vi "gimbale.vi"(11 "GIMBAL":refnum<visa-resource-name>) -> ()   [LabVIEW 2014]
uses:
  <vilib>/Instr/_visa.llb/VISA Configure Serial Port (Instr).vi
panel:
  in  "GÓRA 3":bool caption="GÓRA"
  in  "Dӣ 3":bool caption="Dӣ"
  in  "PRAWO 3":bool caption="PRAWO"
  in  "LEWO 3":bool caption="LEWO"
  in  "LEWO 2":bool caption="LEWO"
  in  "PRAWO 2":bool caption="PRAWO"
  in  "stop":bool
  in  "Dӣ":bool
  in  "PRAWO":bool
  in  "LEWO":bool
  in  "GÓRA":bool
  # "sterowanie drugim dużym gimbalem\n(skonfigurowany na trzecim adresie*)\n\n*gimbal do skonfigurowania wg polecenia\nna diagramie"
  # "sterowanie gimbalem dużym\n(skonfigurowany na pierwszym adresie)"
  # "sterowanie gimbalem małym\n(skonfigurowany na drugim adresie)"
  # "UWAGA!\nZatrzymywać program STOPem"
  # "Oba gimbale działają na jednym porcie\nUstawić port, na którym widziany jest RS485"
  # "W zależności jak długo jest wciśnięty przycisk, tak długo wykonywany jest ruch gimbalal; \npuszczając przycisk, gimbal przestaje wykonywać ruch; \nnie można wykonywać dwóch ruchów równocześnie na jednym gimbalu;"
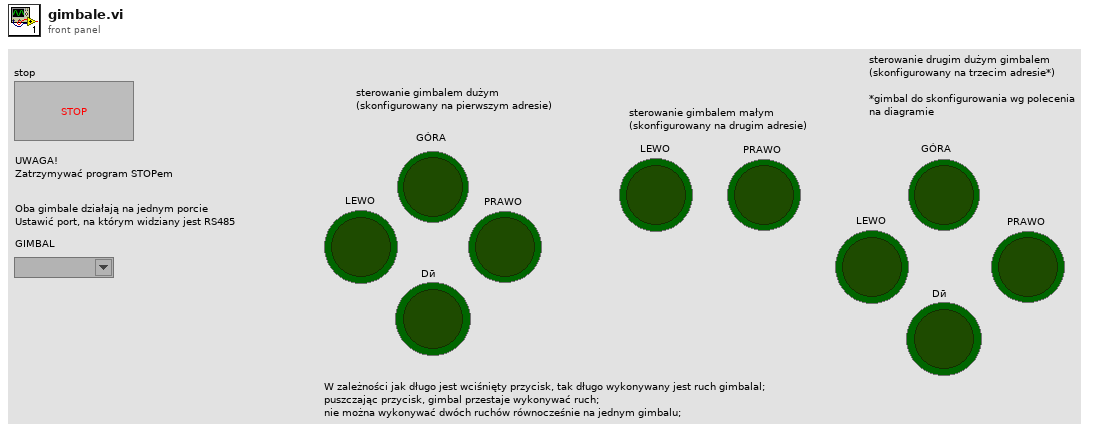
[diagram p1: front panel]
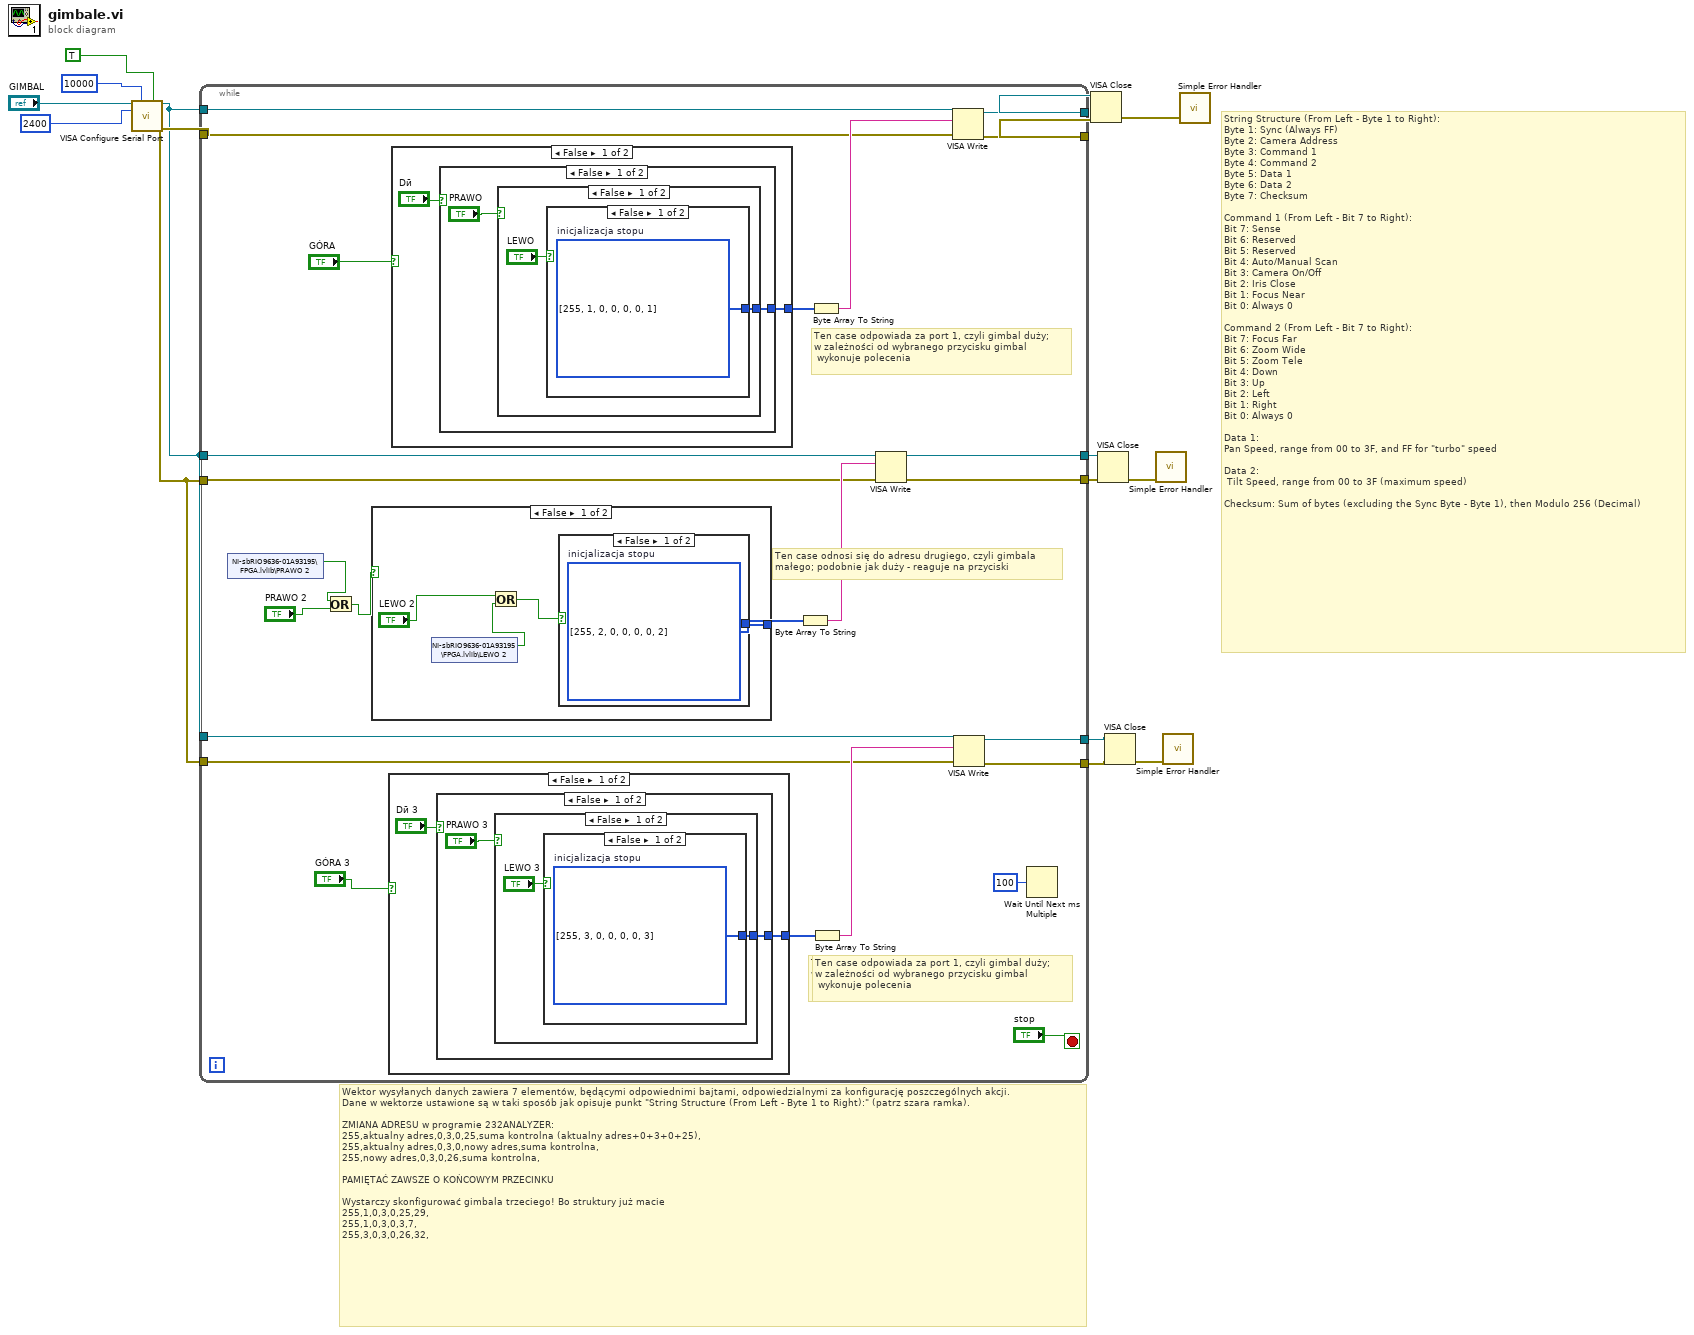
[diagram p0: block diagram]
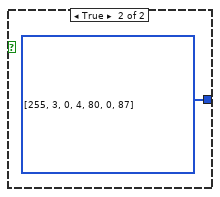
[diagram p2: hidden frame]
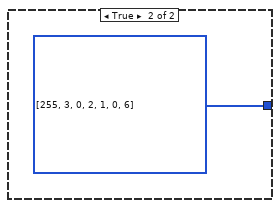
[diagram p3: hidden frame]
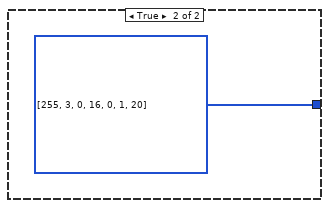
[diagram p4: hidden frame]
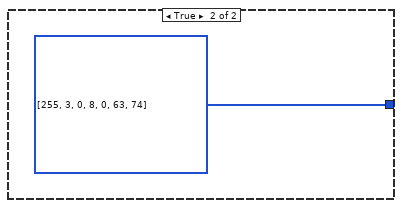
[diagram p5: hidden frame]
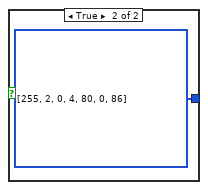
[diagram p6: hidden frame]
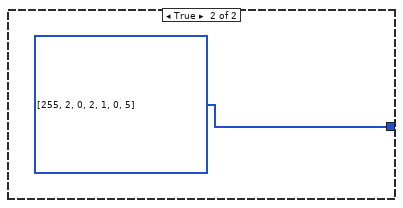
[diagram p7: hidden frame]
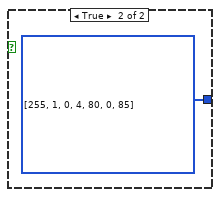
[diagram p8: hidden frame]
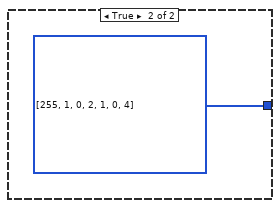
[diagram p9: hidden frame]
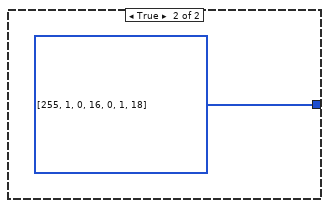
[diagram p10: hidden frame]
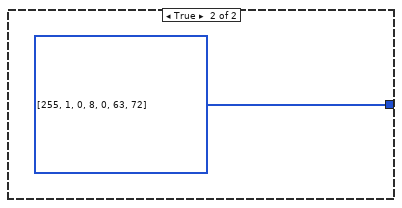
[diagram p11: hidden frame]
diagram:
  # "Wektor wysyłanych danych zawiera 7 elementów, będącymi odpowiednimi bajtami, odpowiedzialnymi za konfigurację poszczególnych akcji.\nDane w wektorze ustawione są w taki sposób jak opisuje punkt \"String Structure (From Left - Byte 1 to Right):\" (patrz szara ramka).\n\nZMIANA ADRESU w programie 232ANALYZER:\n255,aktualny adres,0,3,0,25,suma kontrolna (aktualny adres+0+3+0+25),\n255,aktualny adres,0,3,0,nowy adres,suma kontrolna,\n255,nowy adres,0,3,0,26,suma kontrolna,\n\nPAMIĘTAĆ ZAWSZE O KOŃCOWYM PRZECINKU\n\nWystarczy skonfigurować gimbala trzeciego! Bo struktury już macie\n255,1,0,3,0,25,29,\n255,1,0,3,0,3,7,\n255,3,0,3,0,26,32,"
  # "String Structure (From Left - Byte 1 to Right):\nByte 1: Sync (Always FF)\nByte 2: Camera Address\nByte 3: Command 1\nByte 4: Command 2\nByte 5: Data 1\nByte 6: Data 2\nByte 7: Checksum\n\nCommand 1 (From Left - Bit 7 to Right):\nBit 7: Sense\nBit 6: Reserved\nBit 5: Reserved\nBit 4: Auto/Manual Scan\nBit 3: Camera On/Off\nBit 2: Iris Close\nBit 1: Focus Near\nBit 0: Always 0\n\nCommand 2 (From Left - Bit 7 to Right):\nBit 7: Focus Far\nBit 6: Zoom Wide\nBit 5: Zoom Tele\nBit 4: Down\nBit 3: Up\nBit 2: Left\nBit 1: Right\nBit 0: Always 0\n\nData 1:\nPan Speed, range from 00 to 3F, and FF for \"turbo\" speed\n\nData 2:\n Tilt Speed, range from 00 to 3F (maximum speed)\n\nChecksum: Sum of bytes (excluding the Sync Byte - Byte 1), then Modulo 256 (Decimal)"
  n1 = call-poly "VISA Configure Serial Port"("VISA resource name"="GIMBAL", "timeout (10sec)"=u32 10000, "Enable Termination\nChar (T)"=TRUE ("Enable Termination\nChar (T)"), "baud rate (9600)"=u32 2400) -> ("VISA resource name out"=w1:refnum<visa-resource-name>, "error out"=w2:errorcluster)  [unwired: 10 in]
  n2 = while {
    tunnel: w2 -> [w37]
    tunnel: [w36] -> w10
    tunnel: w1 -> [w35]
    tunnel: [w34] -> w9
    tunnel: [w30] -> w7
    tunnel: [w29] -> w6
    tunnel: w1 -> [w28]
    tunnel: w2 -> [w27]
    tunnel: [w25] -> w4
    tunnel: [w24] -> w3
    tunnel: w2 -> [w23]
    tunnel: w1 -> [w22]
    stop <- "stop" stop-if-true
    # "Ten case odpowiada za port 3, czyli gimbal duży;\nw zależności od wybranego przycisku gimbal\n wykonuje polecenia"
    # "Ten case odpowiada za port 1, czyli gimbal duży;\nw zależności od wybranego przycisku gimbal\n wykonuje polecenia"
    # "Ten case odnosi się do adresu drugiego, czyli gimbala \nmałego; podobnie jak duży - reaguje na przyciski"
    # "Ten case odpowiada za port 1, czyli gimbal duży;\nw zależności od wybranego przycisku gimbal\n wykonuje polecenia"
    n3 = shared-variable "NI-sbRIO9636-01A93195\\FPGA.lvlib\\PRAWO 2"() -> (w16:bool)  [unwired: 1 in, 1 out]
    n4 = Or(x=w16, y="PRAWO 2") -> (x .or. y?=w18:bool)
    n5 = case shown="False" w18 {
      tunnel: [w55 u8[] [255, 2, 0, 2, 1, 0, 5] ("inicjalizacja stopu")] -> w32
      frame False {
        n6 = shared-variable "NI-sbRIO9636-01A93195\\FPGA.lvlib\\LEWO 2"() -> (w52:bool)  [unwired: 1 in, 1 out]
        n7 = Or(x="LEWO 2", y=w52) -> (x .or. y?=w54:bool)
        n8 = case shown="False" w54 {
          tunnel: [w56 u8[] [255, 2, 0, 4, 80, 0, 86] ("inicjalizacja stopu")] -> w55
          frame False {
            w56 = u8[] [255, 2, 0, 0, 0, 0, 2]  # inicjalizacja stopu
          }
          frame True {
          }
        }
      }
      frame True {
      }
    }
    n9 = case shown="False" "GÓRA 3" {
      tunnel: [w41 u8[] [255, 3, 0, 8, 0, 63, 74] ("inicjalizacja stopu")] -> w20
      frame False {
        n10 = case shown="False" "Dӣ 3" {
          tunnel: [w43 u8[] [255, 3, 0, 16, 0, 1, 20] ("inicjalizacja stopu")] -> w41
          frame False {
            n11 = case shown="False" "PRAWO 3" {
              tunnel: [w46 u8[] [255, 3, 0, 2, 1, 0, 6] ("inicjalizacja stopu")] -> w43
              frame False {
                n12 = case shown="False" "LEWO 3" {
                  tunnel: [w47 u8[] [255, 3, 0, 4, 80, 0, 87] ("inicjalizacja stopu")] -> w46
                  frame False {
                    w47 = u8[] [255, 3, 0, 0, 0, 0, 3]  # inicjalizacja stopu
                  }
                  frame True {
                  }
                }
              }
              frame True {
              }
            }
          }
          frame True {
          }
        }
      }
      frame True {
      }
    }
    n13 = case shown="False" "GÓRA" {
      tunnel: [w59 u8[] [255, 1, 0, 8, 0, 63, 72] ("inicjalizacja stopu")] -> w39
      frame False {
        n14 = case shown="False" "Dӣ" {
          tunnel: [w61 u8[] [255, 1, 0, 16, 0, 1, 18] ("inicjalizacja stopu")] -> w59
          frame False {
            n15 = case shown="False" "PRAWO" {
              tunnel: [w64 u8[] [255, 1, 0, 2, 1, 0, 4] ("inicjalizacja stopu")] -> w61
              frame False {
                n16 = case shown="False" "LEWO" {
                  tunnel: [w65 u8[] [255, 1, 0, 4, 80, 0, 85] ("inicjalizacja stopu")] -> w64
                  frame False {
                    w65 = u8[] [255, 1, 0, 0, 0, 0, 1]  # inicjalizacja stopu
                  }
                  frame True {
                  }
                }
              }
              frame True {
              }
            }
          }
          frame True {
          }
        }
      }
      frame True {
      }
    }
    n17 = Byte Array To String(unsigned byte array=w32) -> (string=w31:string)
    n18 = Byte Array To String(unsigned byte array=w39) -> (string=w38:string)
    n19 = Byte Array To String(unsigned byte array=w20) -> (string=w26:string)
    n20 = VISA Write(VISA resource name=w28, write buffer=w31, error in (no error)=w27) -> (VISA resource name out=w29:refnum<visa-resource-name>, error out=w30:errorcluster)  [unwired: 1 out]
    n21 = VISA Write(VISA resource name=w35, write buffer=w38, error in (no error)=w37) -> (VISA resource name out=w34:refnum<visa-resource-name>, error out=w36:errorcluster)  [unwired: 1 out]
    n22 = VISA Write(VISA resource name=w22, write buffer=w26, error in (no error)=w23) -> (VISA resource name out=w25:refnum<visa-resource-name>, error out=w24:errorcluster)  [unwired: 1 out]
    n23 = Wait Until Next ms Multiple(millisecond multiple=u32 100) -> ()  [unwired: 1 out]
  }
  n24 = VISA Close(VISA resource name=w9, error in (no error)=w10) -> (error out=w11:errorcluster)
  n25 = VISA Close(VISA resource name=w6, error in (no error)=w7) -> (error out=w8:errorcluster)
  n26 = VISA Close(VISA resource name=w4, error in (no error)=w3) -> (error out=w5:errorcluster)
  n27 = call <vilib>:"Simple Error Handler.vi"("error in (no error)"=w8) -> ()  [unwired: 4 in, 5 out]
  n28 = call <vilib>:"Simple Error Handler.vi"("error in (no error)"=w5) -> ()  [unwired: 4 in, 5 out]
  n29 = call <vilib>:"Simple Error Handler.vi"("error in (no error)"=w11) -> ()  [unwired: 4 in, 5 out]
